vi "DP-Create Queue Data.vi"(0 "State in":T1, 5 "Parameters":T2, 7 "Right":string, 9 "Left":string) -> (4 "State out":T1, 6 "run":i32, 8 "data":T5, 15 "error out":errorcluster)   [LabVIEW 2020]
uses:
  Typedefs/DP-Queue Data.ctl
  Typedefs/DP-Parameters.ctl
  Typedefs/DP-Stimulus Params.ctl
  Typedefs/DP-Response Params.ctl
  CFTS VIs/CFTS-Experiment State.ctl
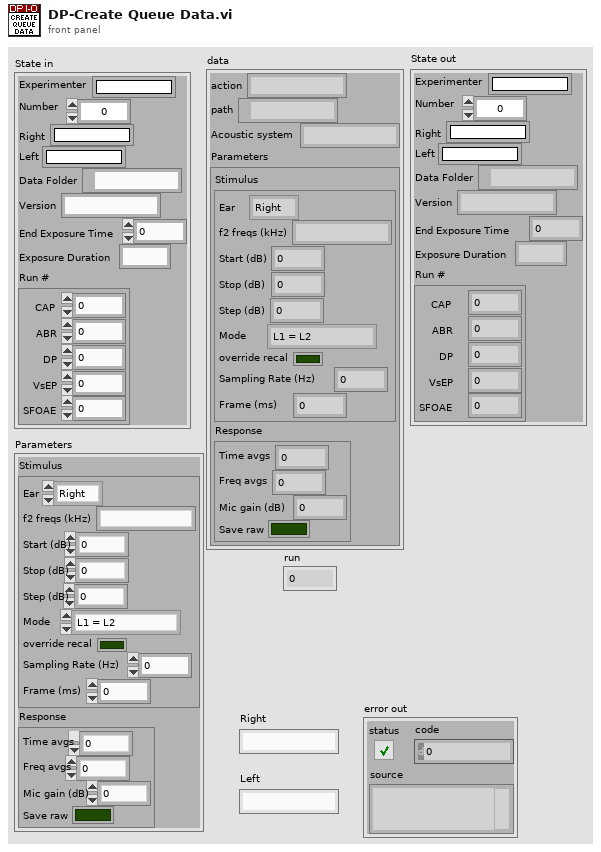
[diagram p1: front panel]
types:
  T1 = typedef "CFTS-Experiment State.ctl" = cluster{"Experimenter":string, "Number":u32, "Right":string, "Left":string, "Data Folder":path, "Version":string, "End Exposure Time":dbl, "Exposure Duration":string, "Run #":cluster{"CAP":i32, "ABR":i32, "DP":i32, "VsEP":i32, "SFOAE":i32}}
  T2 = typedef "DP-Parameters.ctl" = cluster{"Stimulus":T3, "Response":T4}
  T3 = typedef "DP-Stimulus Params.ctl" = cluster{"Ear":enum16{"Right", "Left"}, "f2 freqs (kHz)":string, "Start (dB)":dbl, "Stop (dB)":dbl, "Step (dB)":dbl, "Mode":enum16{"L1 = L2", "L1 = L2 + 10 dB"}, "override recal":bool, "Sampling Rate (Hz)":dbl, "Frame (ms)":dbl}
  T4 = typedef "DP-Response Params.ctl" = cluster{"Time avgs":i32, "Freq avgs":i32, "Mic gain (dB)":dbl, "Save raw":bool}
  T5 = typedef "DP-Queue Data.ctl" = cluster{"action":string, "path":path, "Acoustic system":string, "Parameters":T2}
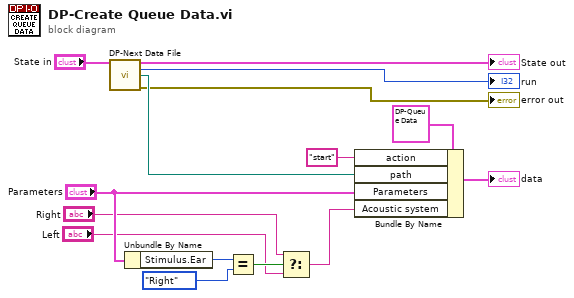
[diagram p0: block diagram]
diagram:
  n1 = call "DP-Next Data File.vi"("State in"="State in") -> ("State out"=→"State out":T1, "run"=→"run":i32, "data path"=w11:path, "error out"=→"error out":errorcluster)  [unwired: 11 in]
  n2 = Unbundle By Name("Parameters") -> ("Stimulus.Ear"=w7:enum16{"Right", "Left"})
  n3 = Equal?(x=w7, y=enum16{"Right", "Left"}."Right") -> (x = y?=w4:bool)
  n4 = Select(t="Right", s=w4, f="Left") -> (s? t:f=w3:string)
  n5 = Bundle By Name(cluster=T5 {"action"="", "path"=path "", "Acoustic system"="", "Parameters"={"Stimulus"={"Ear"=enum."Right", "f2 freqs (kHz)"="", "Start (dB)"=0.0, "Stop (dB)"=0.0, "Step (dB)"=0.0, "Mode"=enum."L1 = L2", "override recal"=FALSE, "Sampling Rate (Hz)"=0.0, "Frame (ms)"=0.0}, "Response"={"Time avgs"=0, "Freq avgs"=0, "Mic gain (dB)"=0.0, "Save raw"=FALSE}}} ("data"), "action"="start", "path"=w11, "Parameters"="Parameters", "Acoustic system"=w3) -> (→"data":T5)
